vi "IMAQdx Ring Buffer to Processing.vi"() -> ()   [LabVIEW 2018]
doc: "The Sequence VI acquires a sequence of images and displays the images in an image control using high-level acquisition VIs. A sequence is appropriate for applications in which you want to process multiple images."
uses:
  <vilib>/vision/Image Controls.llb/IMAQ Image.ctl
panel:
  out "Code Execution Time":cluster{"second":i32, "minute":i32, "hour":i32}
  out "Estimated Processing Time (ms)":u32
  out "# elements in queue":i32
  out "Barcodes (Barcode Reader 1)":T1(array[cluster]) {"Confidence Level" format="%.2f"; "Barcode Type" items=["Reserved", "Codabar", "Code 39", "Code 93", "Code 128", "EAN 8", "EAN 13", "Interleaved 2 of 5", "MSI", "UPCA", "Pharmacode", "RSS Limited"]; "Bounding Box"."y" format="%.2f"; "Bounding Box"."x" format="%.2f"}
  out "Image Consumer":T2(plugin-control)
  in  "# Of Buffers":i32=5
  in  "stop":bool
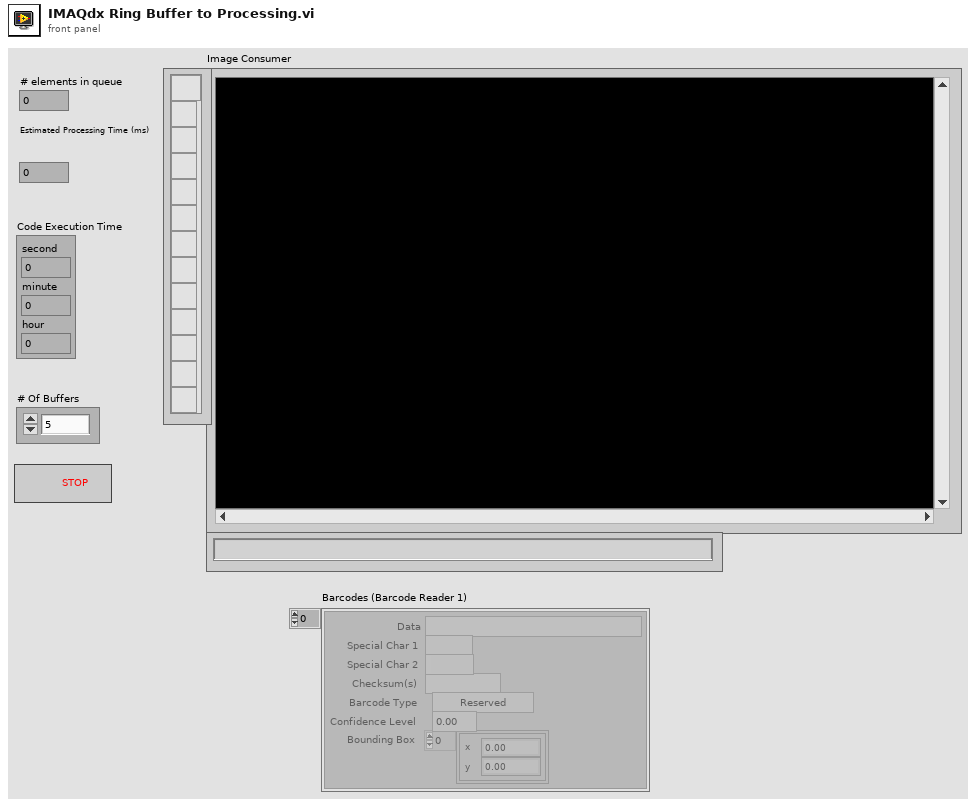
[diagram p1: front panel]
types:
  T1 = cluster{"Data":string, "Special Char 1":string, "Special Char 2":string, "Checksum(s)":string, "Barcode Type":u32, "Confidence Level":sgl, "Bounding Box":cluster{"x":sgl, "y":sgl}[]}[]
  T2 = typedef "IMAQ Image.ctl" = refnum<image>
  T3 = typedef "Image Type" = u32
  T4 = typedef "LVDateTimeRec.ctl" = cluster{"fractional second":dbl, "second":i32, "minute":i32, "hour":i32, "day of month":i32, "month":i32, "year":i32, "day of week":i32, "day of year":i32, "DST":i32}
  T5 = cluster{"Global Rectangle":i32[], "Contours":cluster{"Contour Type":u32, "ROI Type":u32, "Points":i32[]}[]}
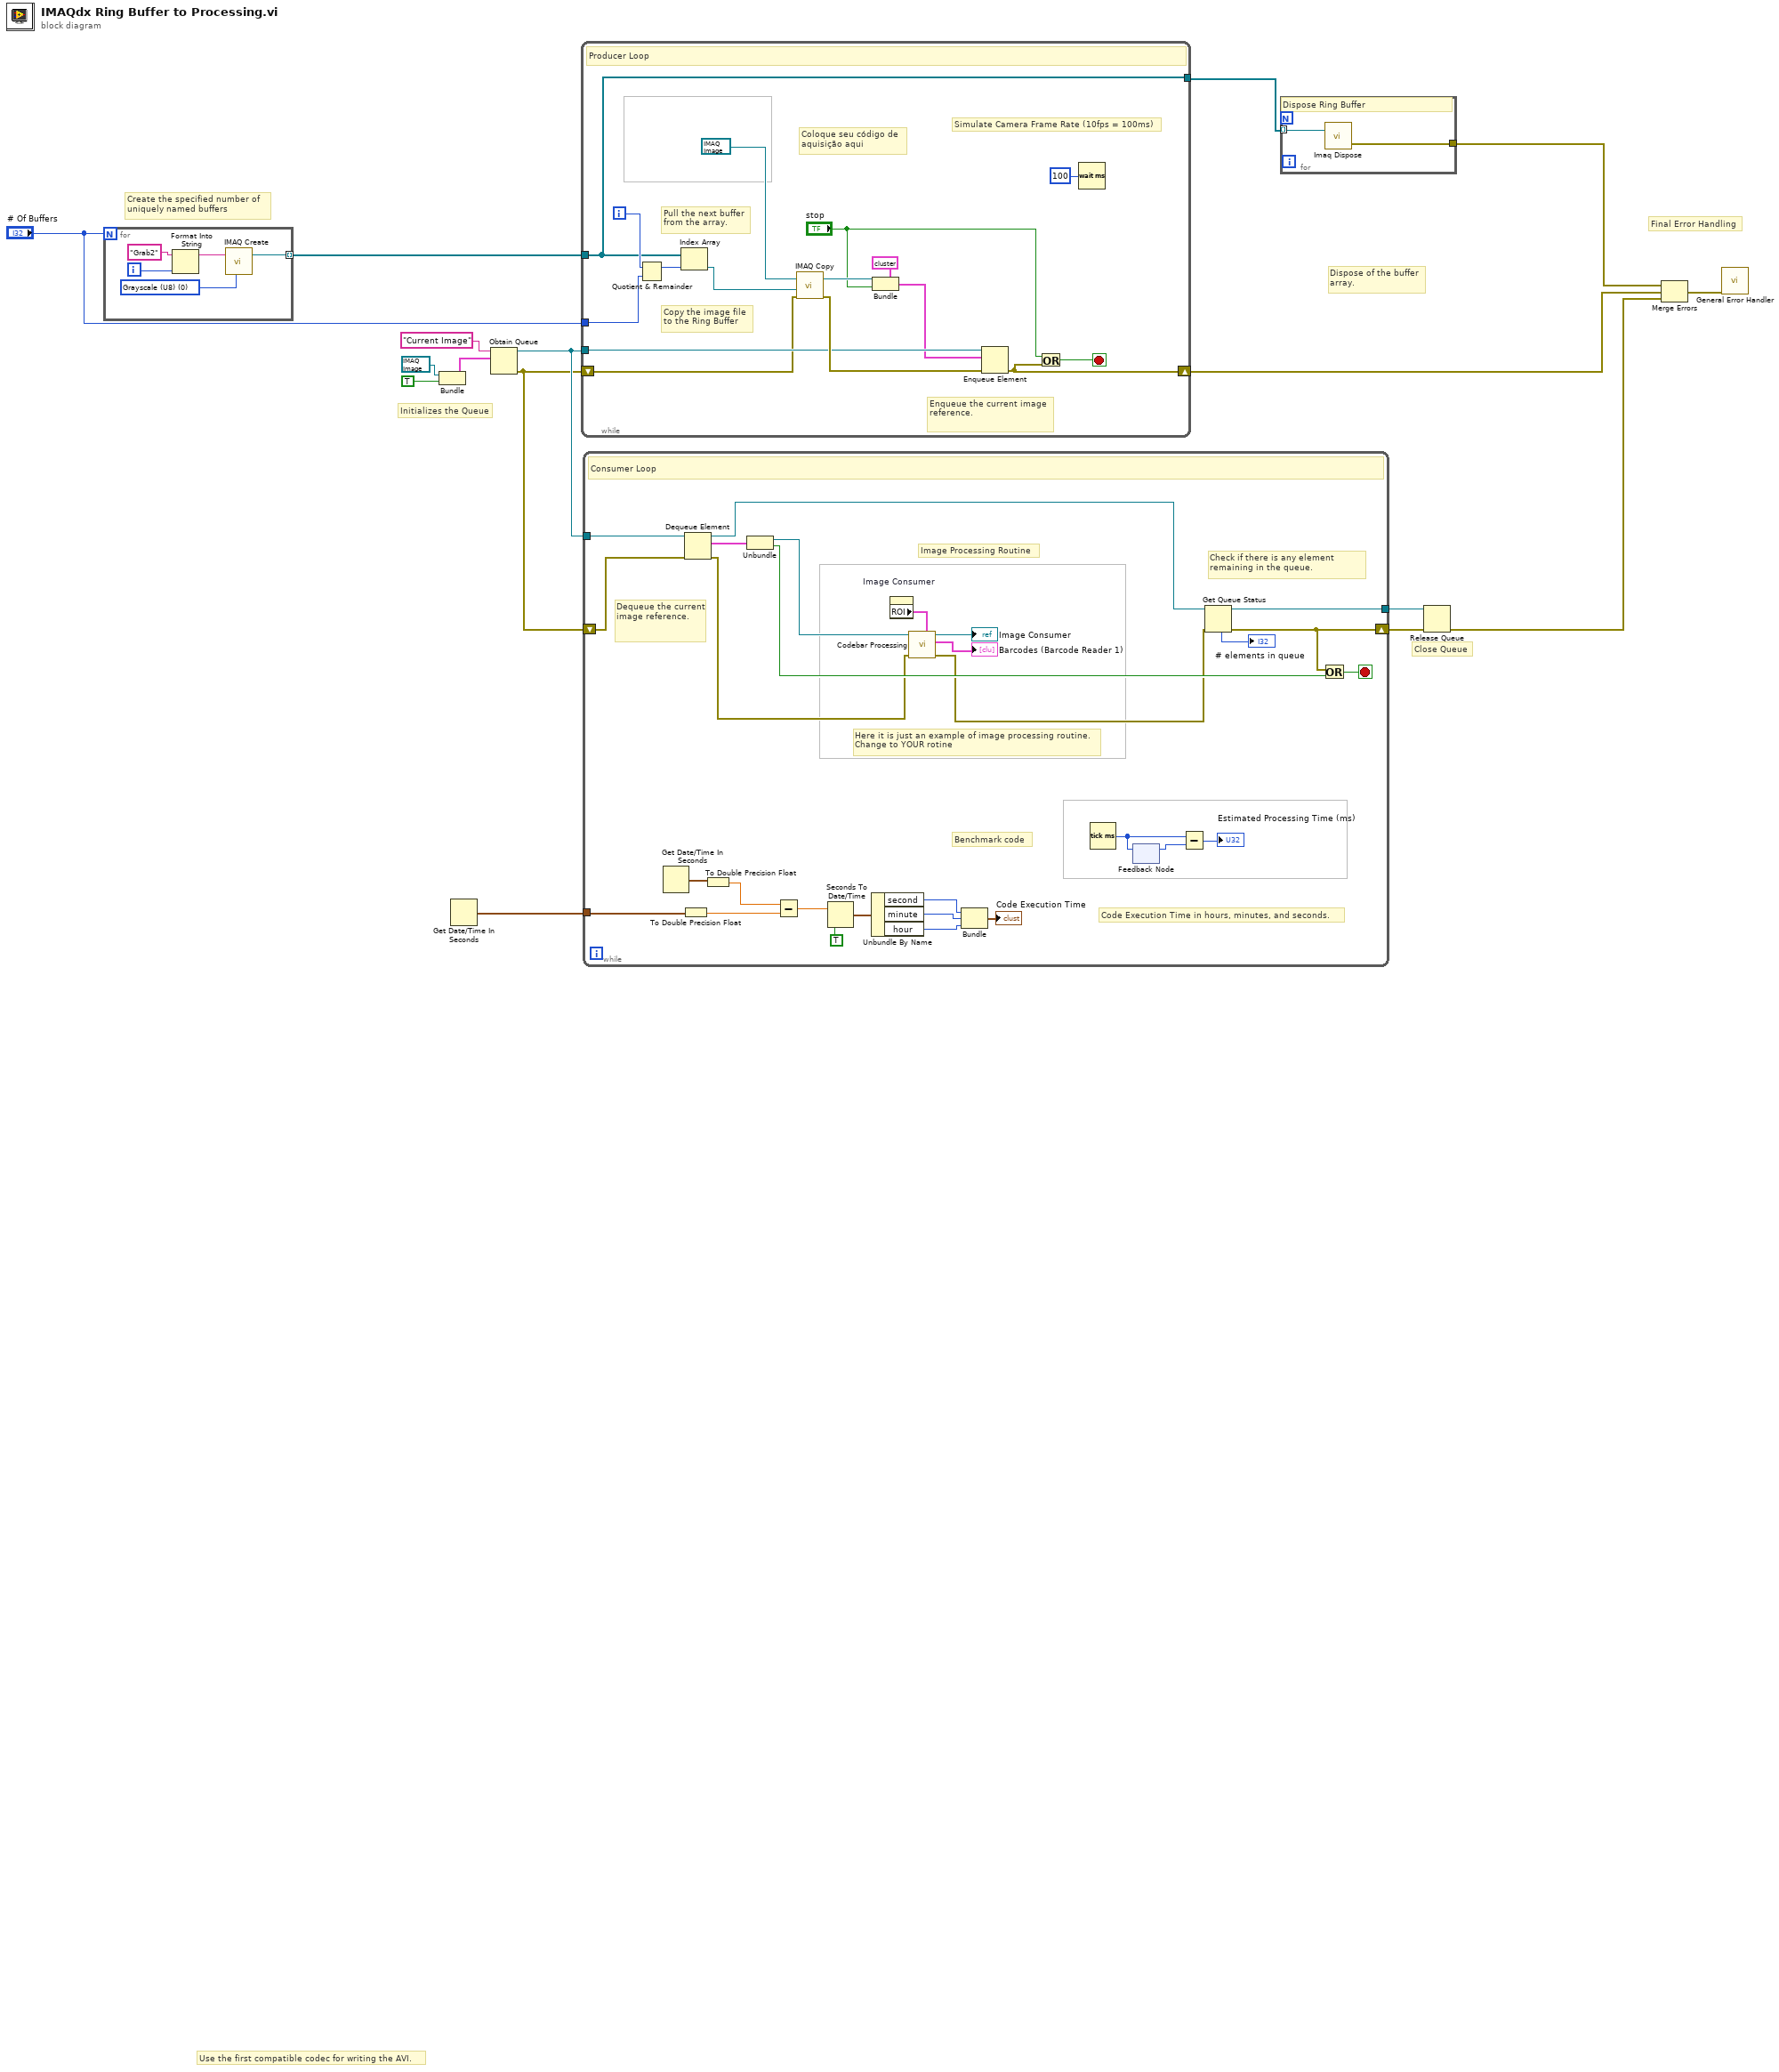
[diagram p0: block diagram]
diagram:
  # "Final Error Handling"
  # "Initializes the Queue"
  # "Close Queue"
  # "Use the first compatible codec for writing the AVI."
  # "Dispose of the buffer\narray."
  # "Create the specified number of \nuniquely named buffers"
  n1 = for {
    N: "# Of Buffers" -> [_]
    tunnel: [w20] -> w4 mode=indexing
    i -> [w19]
    w21 = T3 0 items=["Grayscale (U8)", "Grayscale (I16)", "Grayscale (SGL)", "Complex (CSG)", "RGB (U32)", "HSL (U32)", "RGB (U64)", "Grayscale (U16)"] ("Image Type")
    n2 = Format Into String(initial string="Grab2" ("Image Name"), w19) -> (resulting string=w17:string)  [unwired: 2 in, 1 out]
    n3 = call "IMAQ Create"("Image Name"=w17, "Image Type"=w21) -> ("New Image"=w20:T2)  [unwired: 3 in, 1 out]
  }
  n4 = Bundle("New Image"=T2 refnum, TRUE) -> (w11:cluster{"New Image":T2, bool})  [unwired: 1 in]
  n5 = Get Date/Time In Seconds() -> (seconds since 1Jan1904=w8:timestamp)
  n6 = Obtain Queue(name (unnamed)="Current Image", element data type=w11) -> (queue out=w9:refnum<queue>, error out=w2:errorcluster)  [unwired: 3 in, 1 out]
  n7 = while {
    tunnel: "# Of Buffers" -> [w26]
    tunnel: w4 -> [w23]
    tunnel: w9 -> [w32]
    tunnel: [w23] -> w3
    shift-right: [w33] -> w6
    shift-left: w2 -> [w24]
    i -> [w25]
    stop <- w37 stop-if-true
    # "Copy the image file\nto the Ring Buffer"
    # "Simulate Camera Frame Rate (10fps = 100ms)"
    # "Coloque seu código de\naquisição aqui"
    # "Enqueue the current image reference."
    # "Pull the next buffer\nfrom the array."
    # "Producer Loop"
    n8 = Quotient & Remainder(x=w25, y=w26) -> (x-y*floor(x/y)=w36:i32)  [unwired: 1 out]
    n9 = Index Array(array=w23, index=w36) -> (element=w35:T2)
    n10 = call "IMAQ Copy"("error in (no error)"=w24, "Image Dst"=w35, "Image Src"=T2 refnum ("element")) -> ("error out"=w34:errorcluster, "Image Dst Out"=w31:T2)  [unwired: 3 in]
    n11 = Bundle(cluster=cluster{"New Image":T2, bool} {"New Image"=refnum, FALSE} ("output cluster"), "New Image"=w31, "stop") -> (w28:cluster{"New Image":T2, bool})
    n12 = Enqueue Element(queue=w32, element=w28, error in (no error)=w34) -> (error out=w33:errorcluster)  [unwired: 1 in, 2 out]
    n13 = Or(x="stop", y=w33) -> (x .or. y?=w37:bool)
    n14 = Wait (ms)(milliseconds to wait=u32 100) -> ()  [unwired: 1 out]
  }
  n15 = while {
    tunnel: w9 -> [w65]
    tunnel: [w42] -> w14
    tunnel: w8 -> [w52]
    shift-right: [w39] -> w10
    shift-left: w2 -> [w38]
    stop <- w66 stop-if-true
    # "Here it is just an example of image processing routine.\nChange to YOUR rotine"
    # "Image Processing Routine"
    # "Check if there is any element remaining in the queue."
    # "Benchmark code"
    # "Code Execution Time in hours, minutes, and seconds."
    # "Dequeue the current image reference."
    # "Consumer Loop"
    n16 = Get Date/Time In Seconds() -> (seconds since 1Jan1904=w54:timestamp)
    n17 = To Double Precision Float(number=w52) -> (double precision float=w51:dbl)
    n18 = Dequeue Element(queue=w65, error in (no error)=w38) -> (queue out=w43:refnum<queue>, element=w64:cluster{"New Image":T2, bool}, error out=w41:errorcluster)  [unwired: 1 in, 1 out]
    n19 = To Double Precision Float(number=w54) -> (double precision float=w53:dbl)
    n20 = Unbundle(w64) -> ("New Image"=w62:T2, w58:bool)
    n21 = Subtract(x=w53, y=w51) -> (x-y=w50:dbl)
    n22 = Seconds To Date/Time(time stamp (now)=w50, to UTC (F)=TRUE) -> (date time rec=w48:T4)
    n23 = Unbundle By Name(w48) -> ("second"=w47:i32, "minute"=w46:i32, "hour"=w45:i32)
    n24 = property on="Image Consumer" class="ImageControl"() -> ("ROI"=w60:T5)  [unwired: 2 in, 2 out]
    n25 = call "Codebar Processing.vi"("ROI Descriptor"=w60, "error in"=w41, "Image In"=w62) -> ("error out"=w40:errorcluster, "Barcodes (Barcode Reader 1)"=→"Barcodes (Barcode Reader 1)":T1, "Image Out"=→"Image Consumer":T2)  [unwired: 6 in]
    n26 = Bundle("second"=w47, "minute"=w46, "hour"=w45) -> (→"Code Execution Time":cluster{"second":i32, "minute":i32, "hour":i32})  [unwired: 1 in]
    n27 = Tick Count (ms)() -> (millisecond timer value=w57:u32)
    n28 = feedback-in #1(w57) -> ()
    n29 = feedback #1() -> (w56:u32)  [unwired: 1 in]
    n30 = Subtract(x=w57, y=w56) -> (x-y=→"Estimated Processing Time (ms)":u32)
    n31 = Get Queue Status(queue=w43, error in (no error)=w40) -> (queue out=w42:refnum<queue>, error out=w39:errorcluster, # elements in queue=→"# elements in queue":i32)  [unwired: 1 in, 5 out]
    n32 = Or(x=w39, y=w58) -> (x .or. y?=w66:bool)
  }
  n33 = for {
    tunnel: w3 -> [w68] mode=indexing
    tunnel: [w67] -> w1
    # "Dispose Ring Buffer"
    n34 = call "Imaq Dispose"("Image"=w68) -> ("error out"=w67:errorcluster)  [unwired: 2 in, 3 out]
  }
  n35 = Release Queue(queue=w14, error in (no error)=w10) -> (error out=w5:errorcluster)  [unwired: 1 in, 2 out]
  n36 = Merge Errors(w1, w6, w5) -> (w7:errorcluster)
  n37 = call <vilib>:"General Error Handler.vi"("error in (no error)"=w7) -> ()  [unwired: 2 in, 13 out]
